vi "ximc version.vi"(8 "error in (no error)":errorcluster, 11 "version":string) -> (0 "error out":errorcluster, 3 "version out":string)   [LabVIEW 2012, in "libximc.lvlib"]
doc: "void XIMC_API ximc_version (char* version);"
uses:
  libximc.lvlib
  libximc.dll
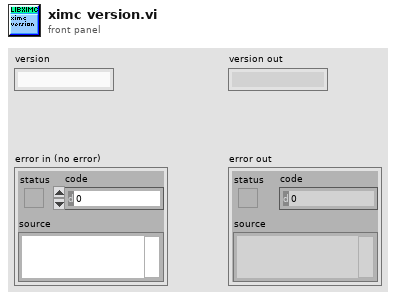
[diagram p1: front panel]
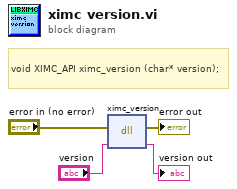
[diagram p0: block diagram]
diagram:
  # "void XIMC_API ximc_version (char* version);"
  n1 = dll-call lib="E:/labview-2.12.1-Labview_12.0/ximcLVx32/libximc.*" fn="ximc_version"(error in="error in (no error)", "version"="version") -> (error out=→"error out":errorcluster, "version"=→"version out":string)  [unwired: 3 in, 1 out]
